vi "MULTTCP2_BlockNetServer.vi"(5 "cmdset":string, 7 "ID":string, 8 "error in (no error)":errorcluster, 9 "notifier In":refnum<notifier>, 10 "messages from sock":refnum<queue>, 11 "listener ID":refnum<k5>) -> (0 "error out":errorcluster)   [LabVIEW 2016]
uses:
  public/vis/coms/TCPSERVER/private/vis/PAN_TCPSERVER_MsgStruct.ctl
  <vilib>/Utility/error.llb/whitespace.ctl
panel:
  in  "ResponseStruct":T1
  out "sock ID":refnum<k5>
  out "stop":bool
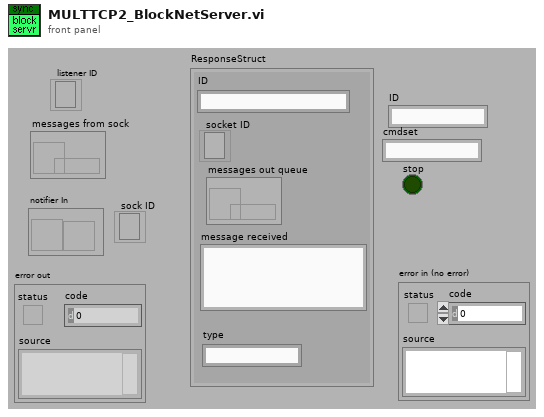
[diagram p1: front panel]
types:
  T1 = typedef "PAN_TCPSERVER_MsgStruct.ctl" = cluster{"ID":string, "socket ID":refnum<k5>, "messages out queue":refnum<queue>, "message received":string, "type":string}
  T2 = enum16{"Standard", "Buffered", "CRLF", "Immediate"}
  T3 = typedef "whitespace.ctl" = u16
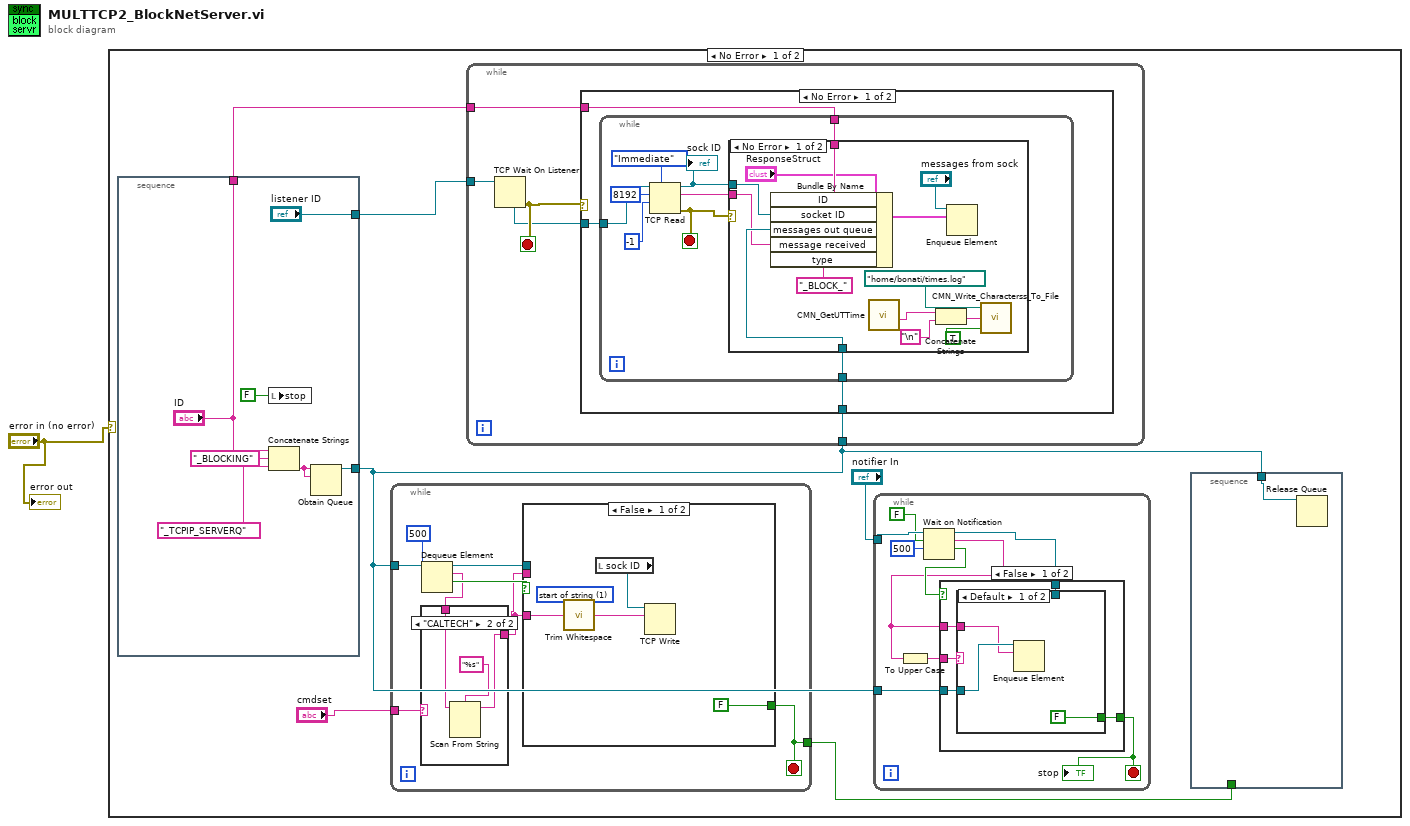
[diagram p0: block diagram]
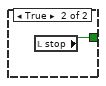
[diagram p3: hidden frame]
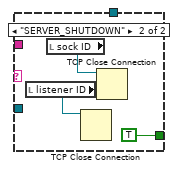
[diagram p4: hidden frame]
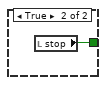
[diagram p5: hidden frame]
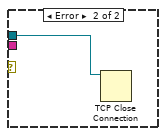
[diagram p6: hidden frame]
diagram:
  n1 = case shown="No Error" "error in (no error)" {
    frame No Error {
      n2 = stacked-sequence {
        tunnel: [w12] -> w3
        tunnel: ["listener ID"] -> w6
        tunnel: ["ID"] -> w5
        frame #0 {
          n3 = local write "stop"(FALSE ("stop")) -> ()
          n4 = Concatenate Strings("ID", "_BLOCKING" ("string"), "_TCPIP_SERVERQ" ("string")) -> (w13:string)
          n5 = Obtain Queue(name (unnamed)=w13, element data type=w13) -> (queue out=w12:refnum<queue>)  [unwired: 3 in, 2 out]
        }
      }
      n6 = while {
        tunnel: w3 -> [w23]
        tunnel: [w19] -> w4
        tunnel: "cmdset" -> [w16]
        stop <- w19 stop-if-true
        n7 = Dequeue Element(queue=w23, timeout in ms (-1)=500) -> (queue out=w22:refnum<queue>, element=w18:string, timed out?=w21:bool)  [unwired: 1 in, 1 out]
        n8 = case shown="\"CALTECH\"" w16 {
          tunnel: w18 -> [w24 w27]
          tunnel: [w24 w25] -> w17
          frame Default {
          }
          frame "CALTECH" {
            n9 = Scan From String(format string="%s", input string=w27) -> (remaining string=w25:string)  [unwired: 2 in, 4 out]
          }
        }
        n10 = case shown="False" w21 {
          tunnel: w17 -> [_ _]
          tunnel: [FALSE w33] -> w19
          tunnel: w22 -> [_ _]
          tunnel: w17 -> [w28 _]
          frame False {
            w29 = T3 1 items=["both", "start of string", "end of string"] ("location (both)")
            n11 = call <vilib>:"Trim Whitespace.vi"("string"=w28, "location (both)"=w29) -> ("trimmed string"=w30:string)
            n12 = local read "sock ID"() -> (w31:refnum<k5>)
            n13 = TCP Write(connection ID=w31, data in=w30) -> ()  [unwired: 1 in, 4 out]
          }
          frame True {
            n14 = local read "stop"() -> (w33:bool)
          }
        }
      }
      n15 = while {
        tunnel: w6 -> [w59]
        tunnel: w3 -> [w56]
        tunnel: w5 -> [w55]
        stop <- w58 stop-if-true
        n16 = TCP Wait On Listener(11:w59) -> (0:w58:errorcluster, 4:w57:refnum<k5>)  [unwired: 1 in, 5 out]
        n17 = case shown="No Error" w58 {
          tunnel: w57 -> [w62 _]
          tunnel: w56 -> [w61 _]
          tunnel: w55 -> [w60 _]
          frame No Error {
            n18 = while {
              tunnel: w62 -> [w71]
              tunnel: w61 -> [w65]
              tunnel: w60 -> [w63]
              stop <- w67 stop-if-true
              n19 = TCP Read(connection ID=w71, bytes to read=8192, 7:T2."Immediate" ("mode (standard)"), 9:-1 ("timeout ms (25000)")) -> (connection ID out=w64:refnum<k5>, data out=w66:string, error out=w67:errorcluster)  [unwired: 1 in]
              "sock ID" <- w64
              n20 = case shown="No Error" w67 {
                tunnel: w66 -> [w80 _]
                tunnel: w65 -> [w82 _]
                tunnel: w64 -> [w84 w85]
                tunnel: w63 -> [w83 _]
                frame No Error {
                  n21 = Bundle By Name(cluster="ResponseStruct", "ID"=w83, "socket ID"=w84, "messages out queue"=w82, "message received"=w80, "type"="_BLOCK_") -> (w77:T1)
                  n22 = call "CMN_GetUTTime.vi"() -> ("str time"=w74:string)  [unwired: 10 out]
                  n23 = Concatenate Strings(w74, "\n") -> (w72:string)
                  n24 = Enqueue Element(queue="messages from sock", element=w77) -> ()  [unwired: 1 in, 4 out]
                  n25 = call "CMN_Write_Characterss_To_File.vi"("append to file? (new file:F)"=TRUE, "character string"=w72, "file path (dialog if empty)"=path "/home/bonati/times.log" ("file (use dialog)")) -> ()  [unwired: 3 out]
                }
                frame Error {
                  n26 = TCP Close Connection(connection ID=w85) -> ()  [unwired: 1 in, 3 out]
                }
              }
            }
          }
          frame Error {
          }
        }
      }
      n27 = while {
        tunnel: "notifier In" -> [w42]
        tunnel: w3 -> [w38]
        stop <- w35 stop-if-true
        n28 = Wait on Notification(notifier=w42, ignore previous (F)=FALSE, timeout in ms (-1)=500) -> (notifier out=w40:refnum<notifier>, notification=w34:string, timed out?=w36:bool)  [unwired: 1 in, 1 out]
        n29 = To Upper Case(1:w34) -> (0:w39:string)
        n30 = case shown="False" w36 {
          tunnel: w40 -> [w47 _]
          tunnel: w39 -> [w46 _]
          tunnel: [w45 w54] -> w35
          tunnel: w38 -> [w44 _]
          tunnel: w34 -> [w43 _]
          frame False {
            n31 = case shown="Default" w46 {
              tunnel: w47 -> [_ _]
              tunnel: [FALSE TRUE] -> w45
              tunnel: w44 -> [w49 _]
              tunnel: w43 -> [w48 _]
              frame Default {
                n32 = Enqueue Element(queue=w49, element=w48) -> ()  [unwired: 1 in, 4 out]
              }
              frame "SERVER_SHUTDOWN" {
                n33 = local read "listener ID"() -> (w51:refnum<k5>)
                n34 = local read "sock ID"() -> (w52:refnum<k5>)
                n35 = TCP Close Connection(connection ID=w51) -> ()  [unwired: 1 in, 3 out]
                n36 = TCP Close Connection(connection ID=w52) -> ()  [unwired: 1 in, 3 out]
              }
            }
          }
          frame True {
            n37 = local read "stop"() -> (w54:bool)
          }
        }
        "stop" <- w35
      }
      n38 = stacked-sequence {
        tunnel: w4 -> [_]
        tunnel: w3 -> [w8]
        frame #0 {
          n39 = Release Queue(queue=w8) -> ()  [unwired: 1 in, 4 out]
        }
      }
    }
    frame Error {
    }
  }
  "error out" <- "error in (no error)"
